vi "UDP IMU9 T2021.vi"(7 "T=last value, F=zero":bool, 8 "Error In":errorcluster, 11 "data in":string) -> (0 "Error Out":errorcluster, 2 "Data Out":T1, 5 "Timeout":bool)   [LabVIEW 2021]
uses:
  IMU data typedef.ctl
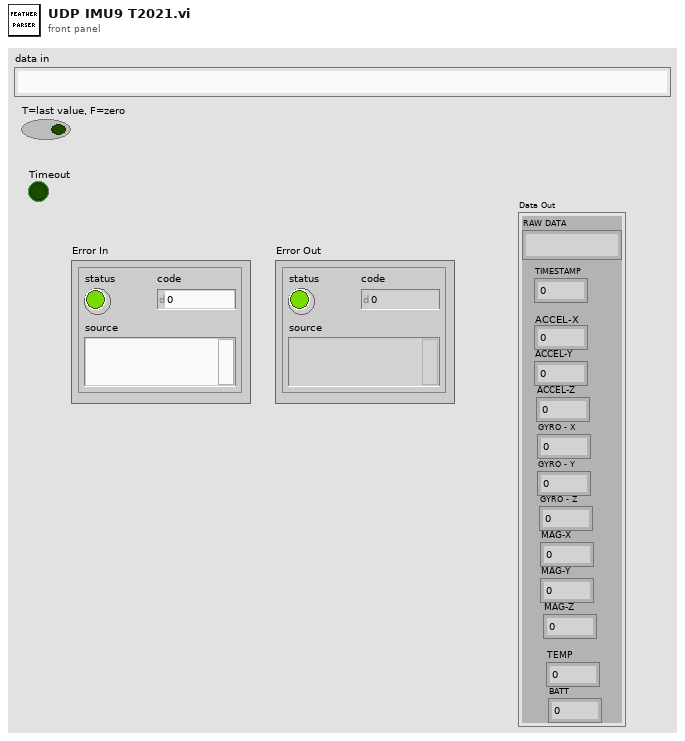
[diagram p1: front panel]
types:
  T1 = typedef "IMU data typedef.ctl" = cluster{"ACCEL-X":dbl, "ACCEL-Y":dbl, "ACCEL-Z":dbl, "GYRO - X":dbl, "GYRO - Y":dbl, "GYRO - Z":dbl, "MAG-Z":dbl, "MAG-Y":dbl, "MAG-X":dbl, "TEMP":dbl, "BATT":dbl, "RAW DATA":string, "TIMESTAMP":dbl}
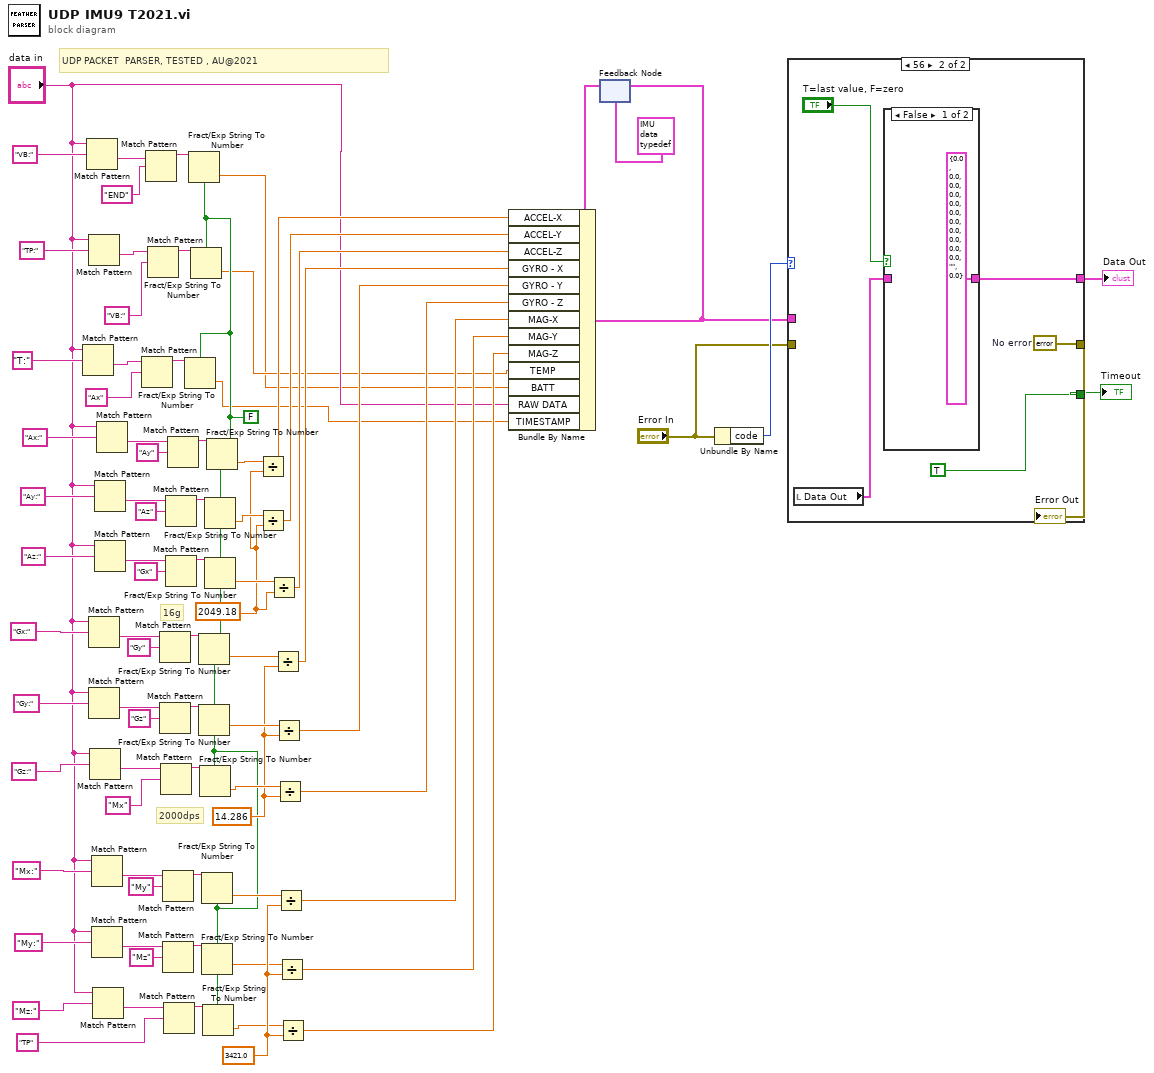
[diagram p0: block diagram]
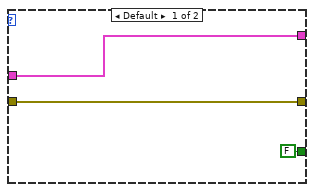
[diagram p2: hidden frame]
diagram:
  w32 = 3421.0 ("y")
  w43 = 14.286 ("y")
  w47 = 2049.18 ("y")
  w16 = FALSE ("use system decimal point (T)")
  # "UDP PACKET  PARSER, TESTED , AU@2021"
  # "2000dps"
  # "16g"
  n1 = Match Pattern(string="data in", regular expression="T:") -> (after substring=w56:string)  [unwired: 1 in, 3 out]
  n2 = Match Pattern(string="data in", regular expression="VB:") -> (after substring=w35:string)  [unwired: 1 in, 3 out]
  n3 = Match Pattern(string="data in", regular expression="TP:") -> (after substring=w37:string)  [unwired: 1 in, 3 out]
  n4 = Match Pattern(string="data in", regular expression="Gx:") -> (after substring=w69:string)  [unwired: 1 in, 3 out]
  n5 = Match Pattern(string="data in", regular expression="Gy:") -> (after substring=w64:string)  [unwired: 1 in, 3 out]
  n6 = Match Pattern(string="data in", regular expression="Gz:") -> (after substring=w61:string)  [unwired: 1 in, 3 out]
  n7 = Match Pattern(string="data in", regular expression="Mx:") -> (after substring=w18:string)  [unwired: 1 in, 3 out]
  n8 = Match Pattern(string="data in", regular expression="My:") -> (after substring=w23:string)  [unwired: 1 in, 3 out]
  n9 = Match Pattern(string="data in", regular expression="Mz:") -> (after substring=w26:string)  [unwired: 1 in, 3 out]
  n10 = Match Pattern(string="data in", regular expression="Ay:") -> (after substring=w77:string)  [unwired: 1 in, 3 out]
  n11 = Match Pattern(string="data in", regular expression="Az:") -> (after substring=w80:string)  [unwired: 1 in, 3 out]
  n12 = Match Pattern(string="data in", regular expression="Ax:") -> (after substring=w72:string)  [unwired: 1 in, 3 out]
  n13 = Match Pattern(string=w56, regular expression="Ax") -> (before substring=w58:string)  [unwired: 1 in, 3 out]
  n14 = Match Pattern(string=w35, regular expression="END") -> (before substring=w39:string)  [unwired: 1 in, 3 out]
  n15 = Match Pattern(string=w37, regular expression="VB:") -> (before substring=w38:string)  [unwired: 1 in, 3 out]
  n16 = Match Pattern(string=w69, regular expression="Gy") -> (before substring=w67:string)  [unwired: 1 in, 3 out]
  n17 = Match Pattern(string=w64, regular expression="Gz") -> (before substring=w66:string)  [unwired: 1 in, 3 out]
  n18 = Match Pattern(string=w61, regular expression="Mx") -> (before substring=w59:string)  [unwired: 1 in, 3 out]
  n19 = Match Pattern(string=w18, regular expression="My") -> (before substring=w20:string)  [unwired: 1 in, 3 out]
  n20 = Match Pattern(string=w23, regular expression="Mz") -> (before substring=w21:string)  [unwired: 1 in, 3 out]
  n21 = Match Pattern(string=w26, regular expression="TP") -> (before substring=w28:string)  [unwired: 1 in, 3 out]
  n22 = Match Pattern(string=w77, regular expression="Az") -> (before substring=w75:string)  [unwired: 1 in, 3 out]
  n23 = Match Pattern(string=w80, regular expression="Gx") -> (before substring=w82:string)  [unwired: 1 in, 3 out]
  n24 = Match Pattern(string=w72, regular expression="Ay") -> (before substring=w74:string)  [unwired: 1 in, 3 out]
  n25 = Fract/Exp String To Number(use system decimal point (T)=w16, string=w58) -> (number=w5:dbl)  [unwired: 2 in, 1 out]
  n26 = Fract/Exp String To Number(use system decimal point (T)=w16, string=w39) -> (number=w2:dbl)  [unwired: 2 in, 1 out]
  n27 = Fract/Exp String To Number(use system decimal point (T)=w16, string=w38) -> (number=w3:dbl)  [unwired: 2 in, 1 out]
  n28 = Fract/Exp String To Number(use system decimal point (T)=w16, string=w67) -> (number=w46:dbl)  [unwired: 2 in, 1 out]
  n29 = Fract/Exp String To Number(use system decimal point (T)=w16, string=w66) -> (number=w45:dbl)  [unwired: 2 in, 1 out]
  n30 = Fract/Exp String To Number(use system decimal point (T)=w16, string=w59) -> (number=w44:dbl)  [unwired: 2 in, 1 out]
  n31 = Fract/Exp String To Number(use system decimal point (T)=w16, string=w20) -> (number=w29:dbl)  [unwired: 2 in, 1 out]
  n32 = Fract/Exp String To Number(use system decimal point (T)=w16, string=w21) -> (number=w30:dbl)  [unwired: 2 in, 1 out]
  n33 = Fract/Exp String To Number(use system decimal point (T)=w16, string=w28) -> (number=w31:dbl)  [unwired: 2 in, 1 out]
  n34 = Fract/Exp String To Number(use system decimal point (T)=w16, string=w75) -> (number=w50:dbl)  [unwired: 2 in, 1 out]
  n35 = Fract/Exp String To Number(use system decimal point (T)=w16, string=w82) -> (number=w48:dbl)  [unwired: 2 in, 1 out]
  n36 = Fract/Exp String To Number(use system decimal point (T)=w16, string=w74) -> (number=w49:dbl)  [unwired: 2 in, 1 out]
  n37 = Divide(x=w49, y=w47) -> (x/y=w14:dbl)
  n38 = Divide(x=w50, y=w47) -> (x/y=w13:dbl)
  n39 = Divide(x=w48, y=w47) -> (x/y=w12:dbl)
  n40 = Divide(x=w46, y=w43) -> (x/y=w11:dbl)
  n41 = Divide(x=w45, y=w43) -> (x/y=w10:dbl)
  n42 = Divide(x=w44, y=w43) -> (x/y=w9:dbl)
  n43 = Divide(x=w29, y=w32) -> (x/y=w8:dbl)
  n44 = Divide(x=w30, y=w32) -> (x/y=w7:dbl)
  n45 = Divide(x=w31, y=w32) -> (x/y=w6:dbl)
  n46 = feedback #1(T1 {"ACCEL-X"=0.0, "ACCEL-Y"=0.0, "ACCEL-Z"=0.0, "GYRO - X"=0.0, "GYRO - Y"=0.0, "GYRO - Z"=0.0, "MAG-Z"=0.0, "MAG-Y"=0.0, "MAG-X"=0.0, "TEMP"=0.0, "BATT"=0.0, "RAW DATA"="", "TIMESTAMP"=0.0} ("Data Out")) -> (w15:T1)
  n47 = Bundle By Name(cluster=w15, "ACCEL-X"=w14, "ACCEL-Y"=w13, "ACCEL-Z"=w12, "GYRO - X"=w11, "GYRO - Y"=w10, "GYRO - Z"=w9, "MAG-X"=w8, "MAG-Y"=w7, "MAG-Z"=w6, "TEMP"=w3, "BATT"=w2, "RAW DATA"="data in", "TIMESTAMP"=w5) -> (w1:T1)
  n48 = feedback-in #1(w1) -> ()
  n49 = Unbundle By Name("Error In") -> ("code"=w54:i32)
  n50 = case shown="56" w54 {
    tunnel: "Error In" -> [w85 _]
    tunnel: [w85 w90] -> w52
    tunnel: [w84 w88] -> w42
    tunnel: w1 -> [w84 _]
    tunnel: [FALSE ("status") TRUE ("status")] -> w51
    frame Default {
    }
    frame 56 {
      w90 = errorcluster {"status"=FALSE, "code"=0, "source"=""}  # No error
      n51 = local read "Data Out"() -> (w87:T1)
      n52 = case shown="False" "T=last value, F=zero" {
        tunnel: [T1 {"ACCEL-X"=0.0, "ACCEL-Y"=0.0, "ACCEL-Z"=0.0, "GYRO - X"=0.0, "GYRO - Y"=0.0, "GYRO - Z"=0.0, "MAG-Z"=0.0, "MAG-Y"=0.0, "MAG-X"=0.0, "TEMP"=0.0, "BATT"=0.0, "RAW DATA"="", "TIMESTAMP"=0.0} ("Data Out") w92] -> w88
        tunnel: w87 -> [_ w92]
        frame False {
        }
        frame True {
        }
      }
    }
  }
  "Error Out" <- w52
  "Data Out" <- w42
  "Timeout" <- w51
